vi "getPosition.vi"(3 "Device":refnum<k24>) -> (1 "GetPOS":dbl)   [LabVIEW 2014]
doc: "André Romero - 2017\nandretec@ifsc.usp.br"
uses:
  C:/UserLabs/Andre/LabView2014-32bits/kinesisTec/Kinesis/Thorlabs.MotionControl.TCube.DCServoCLI.dll
  Kinesis/Thorlabs.MotionControl.TCube.DCServoCLI.dll
  motorsGlobalVar.vi
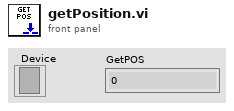
[diagram p1: front panel]
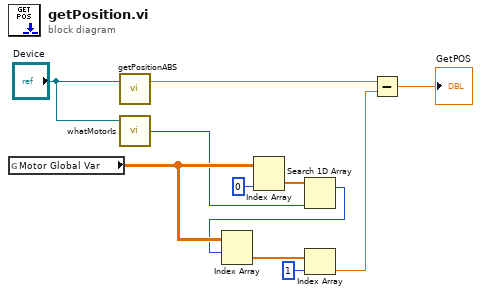
[diagram p0: block diagram]
diagram:
  n1 = global read "motorsGlobalVar.vi" "Motor Global Var"() -> (w7:dbl[][])
  n2 = call "getPositionABS.vi"("Device"="Device") -> ("GetPOS"=w4:dbl)  [unwired: 2 in]
  n3 = call "whatMotorIs.vi"("Device in"="Device") -> ("SerialNumber"=w5:u32)  [unwired: 3 in, 1 out]
  n4 = Index Array(array=w7, index (col)=0 ("disabled index (col)")) -> (element=w10:dbl[])  [unwired: 1 in]
  n5 = Search 1D Array(1D array=w10, element=w5) -> (index of element=w6:i32)  [unwired: 1 in]
  n6 = Index Array(array=w7, index (row)=w6) -> (element=w9:dbl[])  [unwired: 1 in]
  n7 = Index Array(array=w9, index=1) -> (element=w3:dbl)
  n8 = Subtract(x=w4, y=w3) -> (x-y=→"GetPOS":dbl)
